vi "init.vi"(8 "error in (no error)":errorcluster, 10 "Init Data":variant, 11 "Lakeshore 218 in":refnum<class "Lakeshore 218.lvclass">) -> (0 "error out":errorcluster, 2 "Channel List":refnum<class "HK Item.lvclass">[](array[class]), 3 "Lakeshore 218 out":refnum<class "Lakeshore 218.lvclass">)   [LabVIEW 2022 SP3, in "Lakeshore 218.lvclass"]
uses:
  Lakeshore 218.lvclass
  hk-channel-class/hk-channel-class/HK Item/HK Item.lvclass
  Lakeshore 218.lvclass/Lakeshore 218.ctl
  <instrlib>/Lake Shore Cryotronics 218/Lake Shore Cryotronics 218.lvlib
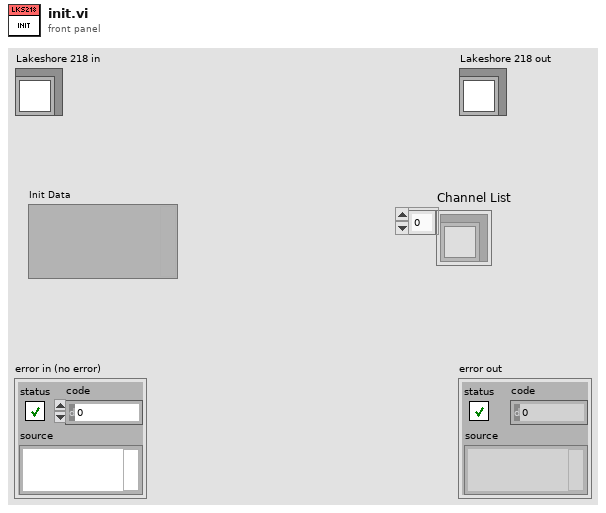
[diagram p1: front panel]
types:
  T1 = typedef "Lakeshore 218.lvclass/Lakeshore 218 cluster Settings.ctl" = cluster{"Port":refnum<visa-resource-name>, "Channel Names":string[], "Ch Enable":bool[]}
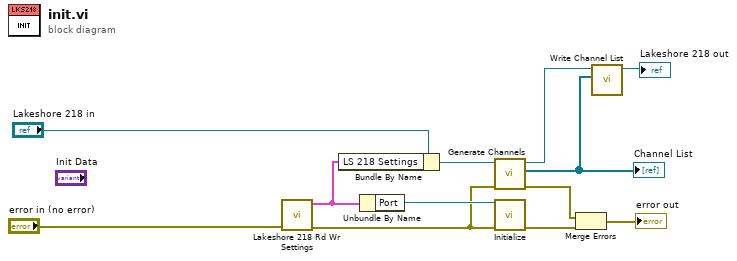
[diagram p0: block diagram]
diagram:
  n1 = call "Lakeshore 218 Rd Wr Settings.vi"("error in (no error)"="error in (no error)") -> ("error out"=w7:errorcluster, "LS 218 Settings"=w10:T1)  [unwired: 9 in]
  n2 = Bundle By Name(cluster="Lakeshore 218 in", "LS 218 Settings"=w10) -> (w8:refnum<class "Lakeshore 218.lvclass">)
  n3 = Unbundle By Name(w10) -> ("Port"=w9:refnum<visa-resource-name>)
  n4 = call-dynamic "Generate Channels.vi"("error in (no error)"=w7, "Lakeshore 218 in"=w8) -> ("error out"=w5:errorcluster, "Channel List"=w1:refnum<class "HK Item.lvclass">[], "Lakeshore 218 out"=w3:refnum<class "Lakeshore 218.lvclass">)  [unwired: 6 in, 1 out]
  "Channel List" <- w1
  n5 = call <instrlib>:"Initialize.vi"("VISA resource name"=w9, "error in (no error)"=w7) -> ("error out"=w6:errorcluster)  [unwired: 12 in, 1 out]
  n6 = Merge Errors(w5, w6) -> (→"error out":errorcluster)
  n7 = call-dynamic "Write Channel List.vi"("Channel List"=w1, "Temp Control in"=w3) -> ("Temp Control out"=→"Lakeshore 218 out":refnum<class "Lakeshore 218.lvclass">)  [unwired: 8 in, 1 out]
